vi "Parse String Arg.vi"(10 "Input String":string) -> (1 "String Arg":string, 2 "Integer Out":i32)   [LabVIEW 2013]
doc: "This sub-VI parses a single string argument and a single integer argument from an input string of the form\n\"state:string:int\". The string argument and integer arguments are then returned."
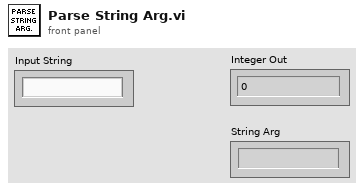
[diagram p1: front panel]
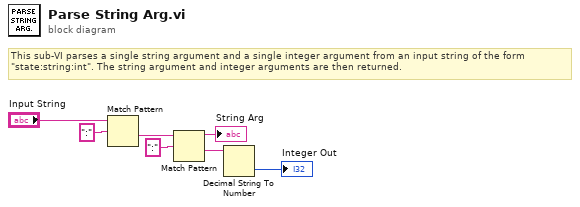
[diagram p0: block diagram]
diagram:
  # "This sub-VI parses a single string argument and a single integer argument from an input string of the form\n\"state:string:int\". The string argument and integer arguments are then returned."
  n1 = Match Pattern(string="Input String", regular expression=":") -> (after substring=w4:string)  [unwired: 1 in, 3 out]
  n2 = Match Pattern(string=w4, regular expression=":") -> (before substring=→"String Arg":string, after substring=w2:string)  [unwired: 1 in, 2 out]
  n3 = Decimal String To Number(string=w2) -> (number=→"Integer Out":i32)  [unwired: 2 in, 1 out]
